vi "Read PathControl.lvclass.vi"(11 "Measurements in":refnum<class "Measurement.lvclass">) -> (2 "PathControl.lvclass":refnum<class "PathControl.lvclass">, 3 "Measurements out":refnum<class "Measurement.lvclass">)   [LabVIEW 2020, in "Measurement.lvclass"]
uses:
  Measurement.lvclass
  Path Control/PathControl.lvclass
  Measurement.lvclass/Measurement.ctl
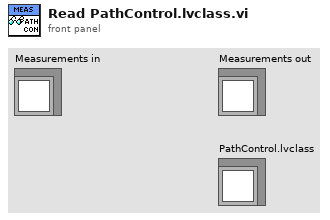
[diagram p1: front panel]
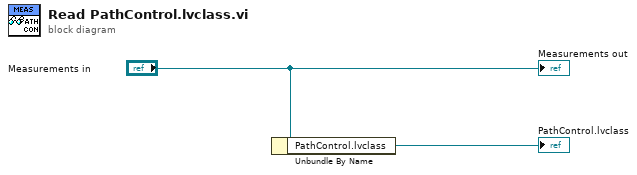
[diagram p0: block diagram]
diagram:
  n1 = Unbundle By Name("Measurements in") -> ("PathControl.lvclass"=→"PathControl.lvclass":refnum<class "PathControl.lvclass">)
  "Measurements out" <- "Measurements in"
